vi "Send BMS Telemetry.vi"   [LabVIEW 2015]
uses:
  Global Data.vi
types:
  T1 = typedef "BMS Telemetry.ctl" = cluster{"bBMSIgnition":bool, "bBMSChargerMains":bool, "bBMSFastCharge":bool, "bBMSChargerEnabled":bool, "eBMSCarState":enum16{"Off", "On, Not Charging", "Charging", "Charging Finished", "Charging Error"}, "eBMSChargingState":enum16{"Disconnected", "Pre-charging", "Main Charging", "Balancing", "Charging Finished OK", "Charging Error"}, "tBMSChargeStage":u16, "eBMSLastChargeError":enum16{"No Error", "No Cell Communication", "No Cell Communication - Non CAN Charger", "Maximum charging stage duration expired", "Cell Communication Lost during Charge", "Cannot set balancing voltage", "Cell temps too high", "No Comms so can't determine temp", "# of Cells Mismatch", "Cells Overvoltage", "Cell Protection Event occured."}, "NBMSNumCells":u8, "bBMSUnderVProtection":bool, "bBMSOverVProtection":bool, "bBMSOverTProtection":bool, "bBMSLeakageProtection":bool, "bBMSNoCellCommsError":bool, "bBMSLowVReduction":bool, "bBMSHighTReduction":bool, "VCellMin":dbl, "VCellMax":dbl, "VCellMean":dbl, "VTotal":dbl, "TCellMin":dbl, "TCellMax":dbl, "TCellMean":dbl, "VCells":cluster{"[51]":dbl, "[53]":dbl, "[54]":dbl, "[55]":dbl, "[56]":dbl, "[57]":dbl, "[58]":dbl, "[59]":dbl, "[60]":dbl, "[61]":dbl, "[62]":dbl, "[63]":dbl, "[64]":dbl, "[65]":dbl, "[66]":dbl, "[67]":dbl, "[34]":dbl, "[35]":dbl, "[36]":dbl, "[37]":dbl, "[38]":dbl, "[39]":dbl, "[40]":dbl, "[41]":dbl, "[42]":dbl, "[43]":dbl, "[44]":dbl, "[45]":dbl, "[46]":dbl, "[47]":dbl, "[48]":dbl, "[49]":dbl, "[50]":dbl, "[17]":dbl, "[18]":dbl, "[19]":dbl, "[20]":dbl, "[21]":dbl, "[22]":dbl, "[23]":dbl, "[24]":dbl, "[25]":dbl, "[26]":dbl, "[27]":dbl, "[28]":dbl, "[29]":dbl, "[30]":dbl, "[31]":dbl, "[32]":dbl, "[33]":dbl, "[0]":dbl, "[1]":dbl, "[2]":dbl, "[3]":dbl, "[4]":dbl, "[5]":dbl, "[6]":dbl, "[7]":dbl, "[8]":dbl, "[9]":dbl, "[10]":dbl, "[11]":dbl, "[12]":dbl, "[13]":dbl, "[14]":dbl, "[15]":dbl, "[16]":dbl, "[52] 2":dbl}, "TBMSCells":cluster{"[55]":dbl, "[56]":dbl, "[57]":dbl, "[58]":dbl, "[59]":dbl, "[60]":dbl, "[61]":dbl, "[62]":dbl, "[63]":dbl, "[64]":dbl, "[65]":dbl, "[66]":dbl, "[67]":dbl, "[68]":dbl, "[69]":dbl, "[70]":dbl, "[17]":dbl, "[38]":dbl, "[39]":dbl, "[40]":dbl, "[41]":dbl, "[42]":dbl, "[43]":dbl, "[44]":dbl, "[45]":dbl, "[46]":dbl, "[47]":dbl, "[48]":dbl, "[49]":dbl, "[50]":dbl, "[51]":dbl, "[52]":dbl, "[53]":dbl, "[54]":dbl, "[21]":dbl, "[22]":dbl, "[23]":dbl, "[24]":dbl, "[25]":dbl, "[26]":dbl, "[27]":dbl, "[28]":dbl, "[29]":dbl, "[30]":dbl, "[31]":dbl, "[32]":dbl, "[33]":dbl, "[34]":dbl, "[35]":dbl, "[36]":dbl, "[37]":dbl, "[0]":dbl, "[1]":dbl, "[2]":dbl, "[3]":dbl, "[4]":dbl, "[5]":dbl, "[6]":dbl, "[7]":dbl, "[8]":dbl, "[9]":dbl, "[10]":dbl, "[11]":dbl, "[12]":dbl, "[13]":dbl, "[14]":dbl, "[15]":dbl, "[16]":dbl}, "bChargerConnected":bool, "VChargerSetpoint":dbl, "IChargerSetpoint":dbl, "VChargerActual":dbl, "IChargerActual":dbl, "BCells":cluster{"[51]":dbl, "[52]":dbl, "[53]":dbl, "[54]":dbl, "[55]":dbl, "[56]":dbl, "[57]":dbl, "[58]":dbl, "[59]":dbl, "[60]":dbl, "[61]":dbl, "[62]":dbl, "[63]":dbl, "[64]":dbl, "[65]":dbl, "[66]":dbl, "[67]":dbl, "[34]":dbl, "[35]":dbl, "[36]":dbl, "[37]":dbl, "[38]":dbl, "[39]":dbl, "[40]":dbl, "[41]":dbl, "[42]":dbl, "[43]":dbl, "[44]":dbl, "[45]":dbl, "[46]":dbl, "[47]":dbl, "[48]":dbl, "[49]":dbl, "[50]":dbl, "[17]":dbl, "[18]":dbl, "[19]":dbl, "[20]":dbl, "[21]":dbl, "[22]":dbl, "[23]":dbl, "[24]":dbl, "[25]":dbl, "[26]":dbl, "[27]":dbl, "[28]":dbl, "[29]":dbl, "[30]":dbl, "[31]":dbl, "[32]":dbl, "[33]":dbl, "[0]":dbl, "[1]":dbl, "[2]":dbl, "[3]":dbl, "[4]":dbl, "[5]":dbl, "[6]":dbl, "[7]":dbl, "[8]":dbl, "[9]":dbl, "[10]":dbl, "[11]":dbl, "[12]":dbl, "[13]":dbl, "[14]":dbl, "[15]":dbl, "[16]":dbl}, "bNewVCellMinSample":bool, "Battery Temp":cluster{"[0]":dbl, "[1]":dbl, "[2]":dbl, "[3]":dbl, "[4]":dbl, "[5]":dbl, "[6]":dbl, "[7]":dbl, "[8]":dbl, "[9]":dbl, "[10]":dbl, "[11]":dbl, "[12]":dbl, "[13]":dbl, "[14]":dbl, "[15]":dbl, "[16]":dbl, "[17]":dbl, "[18]":dbl, "[19]":dbl, "[20]":dbl, "[21]":dbl, "[22]":dbl, "[23]":dbl, "[24]":dbl, "[25]":dbl, "[26]":dbl, "[27]":dbl, "[28]":dbl, "[29]":dbl, "[30]":dbl, "[31]":dbl, "[32]":dbl, "[33]":dbl, "[34]":dbl, "[35]":dbl, "[36]":dbl, "[37]":dbl, "[38]":dbl, "[39]":dbl, "[40]":dbl, "[41]":dbl, "[42]":dbl, "[43]":dbl, "[44]":dbl, "[45]":dbl, "[46]":dbl, "[47]":dbl, "[48]":dbl, "[49]":dbl, "[50]":dbl, "[51]":dbl, "[52]":dbl, "[53]":dbl, "[54]":dbl, "[55]":dbl, "[56]":dbl, "[57]":dbl, "[58]":dbl, "[59]":dbl, "[60]":dbl, "[61]":dbl, "[62]":dbl, "[63]":dbl, "[64]":dbl, "[65]":dbl, "[66]":dbl, "[67]":dbl, "[68]":dbl, "[69]":dbl, "[71]":dbl, "[70]":dbl, "[0] 2":dbl, "[1] 2":dbl, "[2] 2":dbl, "[3] 2":dbl, "[4] 2":dbl, "[5] 2":dbl, "[6] 2":dbl, "[7] 2":dbl, "[8] 2":dbl, "[9] 2":dbl, "[10] 2":dbl, "[11] 2":dbl, "[12] 2":dbl, "[13] 2":dbl, "[14] 2":dbl, "[15] 2":dbl, "[16] 2":dbl, "[17] 2":dbl, "[18] 2":dbl, "[19] 2":dbl, "[20] 2":dbl, "[21] 2":dbl, "[22] 2":dbl, "[23] 2":dbl, "[24] 2":dbl, "[25] 2":dbl, "[26] 2":dbl, "[27] 2":dbl, "[28] 2":dbl, "[29] 2":dbl, "[30] 2":dbl, "[31] 2":dbl, "[32] 2":dbl, "[33] 2":dbl, "[34] 2":dbl, "[35] 2":dbl, "[36] 2":dbl, "[37] 2":dbl, "[38] 2":dbl, "[39] 2":dbl, "[40] 2":dbl, "[41] 2":dbl, "[42] 2":dbl, "[43] 2":dbl, "[44] 2":dbl, "[45] 2":dbl, "[46] 2":dbl, "[47] 2":dbl, "[48] 2":dbl, "[49] 2":dbl, "[50] 2":dbl, "[51] 2":dbl, "[52] 3":dbl, "[53] 2":dbl, "[54] 2":dbl, "[55] 2":dbl, "[56] 2":dbl, "[57] 2":dbl, "[58] 2":dbl, "[59] 2":dbl, "[60] 2":dbl, "[61] 2":dbl, "[62] 2":dbl, "[63] 2":dbl, "[64] 2":dbl, "[65] 2":dbl, "[66] 2":dbl, "[67] 2":dbl, "[68]2":dbl, "[69]2":dbl, "[70]2":dbl, "[71]2":dbl, "[0] 3":dbl, "[1] 3":dbl, "[2] 3":dbl, "[3] 3":dbl, "[4] 3":dbl, "[5] 3":dbl, "[6] 3":dbl, "[7] 3":dbl, "[8] 3":dbl, "[9] 3":dbl, "[10] 3":dbl, "[11] 3":dbl, "[12] 3":dbl, "[13] 3":dbl, "[14] 3":dbl, "[15] 3":dbl, "[16] 3":dbl, "[17] 3":dbl, "[18] 3":dbl, "[19] 3":dbl, "[20] 3":dbl, "[21] 3":dbl, "[22] 3":dbl, "[23] 3":dbl, "[24] 3":dbl, "[25] 3":dbl, "[26] 3":dbl, "[27] 3":dbl, "[28] 3":dbl, "[29] 3":dbl, "[30] 3":dbl, "[31] 3":dbl, "[32] 3":dbl, "[33] 3":dbl, "[34] 3":dbl, "[35] 3":dbl, "[36] 3":dbl, "[37] 3":dbl, "[38] 3":dbl, "[39] 3":dbl, "[40] 3":dbl, "[41] 3":dbl, "[42] 3":dbl, "[43] 3":dbl, "[44] 3":dbl, "[45] 3":dbl, "[46] 3":dbl, "[47] 3":dbl, "[48] 3":dbl, "[49] 3":dbl, "[50] 3":dbl, "[51] 3":dbl, "[52] 4":dbl, "[53] 3":dbl, "[54] 3":dbl, "[55] 3":dbl, "[56] 3":dbl, "[57] 3":dbl, "[58] 3":dbl, "[59] 3":dbl, "[60] 3":dbl, "[61] 3":dbl, "[62] 3":dbl, "[63] 3":dbl, "[64] 3":dbl, "[65] 3":dbl, "[66] 3":dbl, "[67] 3":dbl, "[68]3":dbl, "[69]3":dbl, "[70]3":dbl, "[71]3":dbl, "[4] 4":dbl, "[5] 4":dbl, "[6] 4":dbl, "[7] 4":dbl, "[8] 4":dbl, "[9] 4":dbl, "[10] 4":dbl, "[11] 4":dbl, "[12] 4":dbl, "[13] 4":dbl, "[14] 4":dbl, "[15] 4":dbl, "[16] 4":dbl, "[17] 4":dbl, "[18] 4":dbl, "[19] 4":dbl, "[20] 4":dbl, "[21] 4":dbl, "[22] 4":dbl, "[23] 4":dbl, "[24] 4":dbl, "[25] 4":dbl, "[26] 4":dbl, "[27] 4":dbl, "[28] 4":dbl, "[29] 4":dbl, "[30] 4":dbl, "[31] 4":dbl, "[32] 4":dbl, "[33] 4":dbl, "[17] 9":dbl, "[0] 9":dbl, "[51] 8":dbl, "[34] 8":dbl, "[17] 8":dbl, "[0] 8":dbl, "[34] 4":dbl, "[35] 4":dbl, "[36] 4":dbl, "[37] 4":dbl, "[38] 4":dbl, "[39] 4":dbl, "[40] 4":dbl, "[41] 4":dbl, "[42] 4":dbl, "[43] 4":dbl, "[44] 4":dbl, "[45] 4":dbl, "[46] 4":dbl, "[47] 4":dbl, "[48] 4":dbl, "[49] 4":dbl, "[50] 4":dbl, "[34] 9":dbl, "[51] 4":dbl, "[52] 5":dbl, "[53] 4":dbl, "[54] 4":dbl, "[55] 4":dbl, "[56] 4":dbl, "[57] 4":dbl, "[58] 4":dbl, "[59] 4":dbl, "[60] 4":dbl, "[61] 4":dbl, "[62] 4":dbl, "[63] 4":dbl, "[64] 4":dbl, "[65] 4":dbl, "[66] 4":dbl, "[67] 4":dbl, "[51] 9":dbl}, "TBMSMax":dbl, "TBMSMin":dbl, "TBMSMean":dbl}
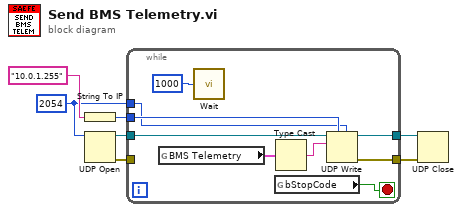
[diagram p0: block diagram]
diagram:
  w2 = u16 2054 ("port")
  n1 = String To IP(1:"10.0.1.255" ("name")) -> (0:w1:u32)
  n2 = UDP Open(11:w2) -> (port=w6:refnum<k16>, 0:w5:errorcluster)  [unwired: 4 in, 1 out]
  n3 = while {
    tunnel: w6 -> [w14]
    tunnel: w5 -> [_]
    tunnel: [w12] -> w4
    tunnel: [w11] -> w3
    tunnel: w1 -> [w10]
    tunnel: w2 -> [w9]
    stop <- w15 stop-if-true
    n4 = global read "Global Data.vi" "BMS Telemetry"() -> (w8:T1)
    n5 = call "Wait"("Count(mSec)"=u32 1000) -> ()  [unwired: 1 out]
    n6 = global read "Global Data.vi" "bStopCode"() -> (w15:bool)
    n7 = Type Cast(x=w8) -> (*(type *) &x=w13:string)  [unwired: 1 in]
    n8 = UDP Write(address=w10, port or service name=w9, connection ID=w14, data in=w13) -> (error out=w11:errorcluster, 3:w12:refnum<k16>)  [unwired: 2 in]
  }
  n9 = UDP Close(connection ID=w4, 8:w3) -> ()  [unwired: 2 out]
